vi "OrdinalEncoder.vi"(8 "error in (no error)":errorcluster caption="entrée d'erreur (pas d'erreur)", 11 "OrdinalEncoder":cluster{"dtype":string}={"dtype"="float"}) -> (0 "error out":errorcluster, 3 "OrdinalEncoder.lvclass":refnum<class "OrdinalEncoder.lvclass">)   [LabVIEW 2020]
doc: "Encode categorical features as an integer array.\n\nThe input to this transformer should be an array-like of integers or strings, denoting the values taken on by categorical (discrete) features. The features are converted to ordinal integers. This results in a single column of integers (0 to n_categories - 1) per feature.\n\n\nParameters : \n\n- dtype : number type, default np.float64\nDesired dtype of output.\n\n\nMethods : \n\n- Fit : Fit the OrdinalEncoder to X.\n\nParameters : X : array-like, shape [n_samples, n_features]\n The data to determine the categories of each feature.\n y : None\n Ignored. \n\n- Fit Transform : Fit to data, then transform it. Fits transformer to X and y with optional parameters fit_params and returns a transformed version of X.\n\nParameters : X : {array-like, sparse matrix, dataframe} of shape (n_samples, n_features)\n y : ndarray of shape (n_samples,), default=None\n Target values.\n\nReturns : X_new : ndarray array of shape (n_samples, n_features_new)\n Transformed array.\n\n\n- Transform : Transform X to ordinal codes.\n\nParameters : X : array-like, shape [n_samples, n_features]\n The data to encode.\n\nReturns : X_out : sparse matrix or a 2-d array\n Transformed input."
uses:
  OrdinalEncoder.lvclass
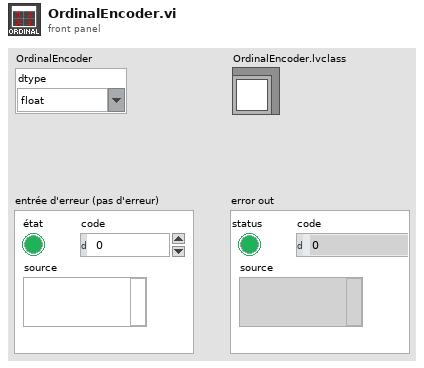
[diagram p1: front panel]
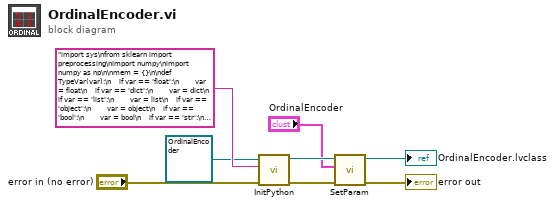
[diagram p0: block diagram]
diagram:
  n1 = call-dynamic "InitPython.vi"("error in (no error)"="error in (no error)", "Python Instruction"="import sys\nfrom sklearn import preprocessing\nimport numpy\nimport numpy as np\n\nmem = {}\n\ndef TypeVar(var):\n    if var == 'float':\n        var = float\n    if var == 'dict':\n        var = dict\n    if var == 'list':\n        var = list\n    if var == 'object':\n        var = object\n    if var == 'bool':\n        var = bool\n    if var == 'str':\n        var = str\n    if var == 'int':\n        var = int\n    return var\n\ndef OrdinalEncoder_Fit(categories, dtype, X, y):\n    X = eval(X)\n    dtype = TypeVar(dtype) \n    if y == 'None' or y == '':\n        y = None\n    else:\n        y = eval(y)\n    try:\n        OrdinalEncoder = preprocessing.OrdinalEncoder(categories, dtype).fit(X, y)\n        mem['FitOrdinalEncoder'] = OrdinalEncoder\n        return str('OK')\n    except:\n        erreur = sys.exc_info()\n        typerr = u\"%s\" % (erreur[0])\n        typerr = typerr[typerr.find(\"'\")+1:typerr.rfind(\"'\")]\n        msgerr = u\"%s\" % (erreur[1])\n        message = str('/!\\\\ {0} : {1}'. format(typerr,msgerr))\n        return message \n    \ndef OrdinalEncoder_FitTransform(categories, dtype, X, y):\n    X = eval(X)\n    dtype = TypeVar(dtype)\n    if y == 'None' or y == '':\n        y = None\n    else:\n        y = eval(y)\n    try:\n        OrdinalEncoder = preprocessing.OrdinalEncoder(categories, dtype).fit_transform(X, y)\n        dtype_func = type(OrdinalEncoder)\n        if dtype_func == numpy.ndarray:\n            OrdinalEncoder = OrdinalEncoder.tolist()\n            return str(OrdinalEncoder) \n        else:\n            Mat = OrdinalEncoder.tocoo()\n            return str(list(zip(Mat.row, Mat.col, Mat.data)))\n    except:\n        erreur = sys.exc_info()\n        typerr = u\"%s\" % (erreur[0])\n        typerr = typerr[typerr.find(\"'\")+1:typerr.rfind(\"'\")]\n        msgerr = u\"%s\" % (erreur[1])\n        message = str('/!\\\\ {0} : {1}'. format(typerr,msgerr))\n        return message \n\ndef OrdinalEncoder_Transform(categories, dtype, X, y):\n    X = eval(X)\n    dtype = TypeVar(dtype)\n    if y == 'None' or y == '':\n        y = None\n    else:\n        y = eval(y)\n    try:\n        OrdinalEncoder = mem['FitOrdinalEncoder'].transform(X)\n        dtype_func = type(OrdinalEncoder)\n        if dtype_func == numpy.ndarray:\n            OrdinalEncoder = OrdinalEncoder.tolist()\n            return str(OrdinalEncoder) \n        else:\n            Mat = OrdinalEncoder.tocoo()\n            return str(list(zip(Mat.row, Mat.col, Mat.data)))\n    except:\n        erreur = sys.exc_info()\n        typerr = u\"%s\" % (erreur[0])\n        typerr = typerr[typerr.find(\"'\")+1:typerr.rfind(\"'\")]\n        msgerr = u\"%s\" % (erreur[1])\n        message = str('/!\\\\ {0} : {1}'. format(typerr,msgerr))\n        return message", "Scikit-learn en entrée"=refnum<class "OrdinalEncoder.lvclass"> refnum ("OrdinalEncoder.lvclass")) -> ("error out"=w4:errorcluster, "Scikit-learn en sortie"=w5:refnum<class "OrdinalEncoder.lvclass">)  [unwired: 7 in]
  n2 = call-dynamic "SetParam.vi"("error in (no error)"=w4, "OrdinalEncoder"="OrdinalEncoder", "OrdinalEncoder.lvclass"=w5) -> ("error out"=→"error out":errorcluster, "OrdinalEncoder.lvclass"=→"OrdinalEncoder.lvclass":refnum<class "OrdinalEncoder.lvclass">)  [unwired: 7 in]
